vi "AutoAdjustYAlxes.vi"(9 "已选信号数组":refnum<vi>, 10 "YaxleNum":i32, 11 "XYGraph输入":refnum<vi>) -> (1 "显示的Y轴数":i32)   [LabVIEW 2015]
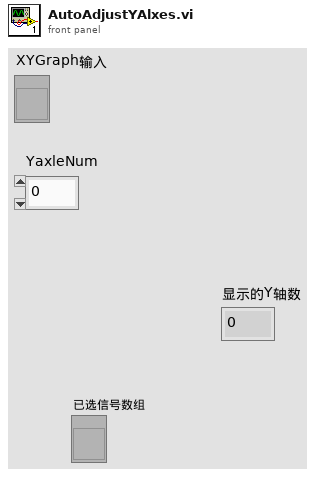
[diagram p1: front panel]
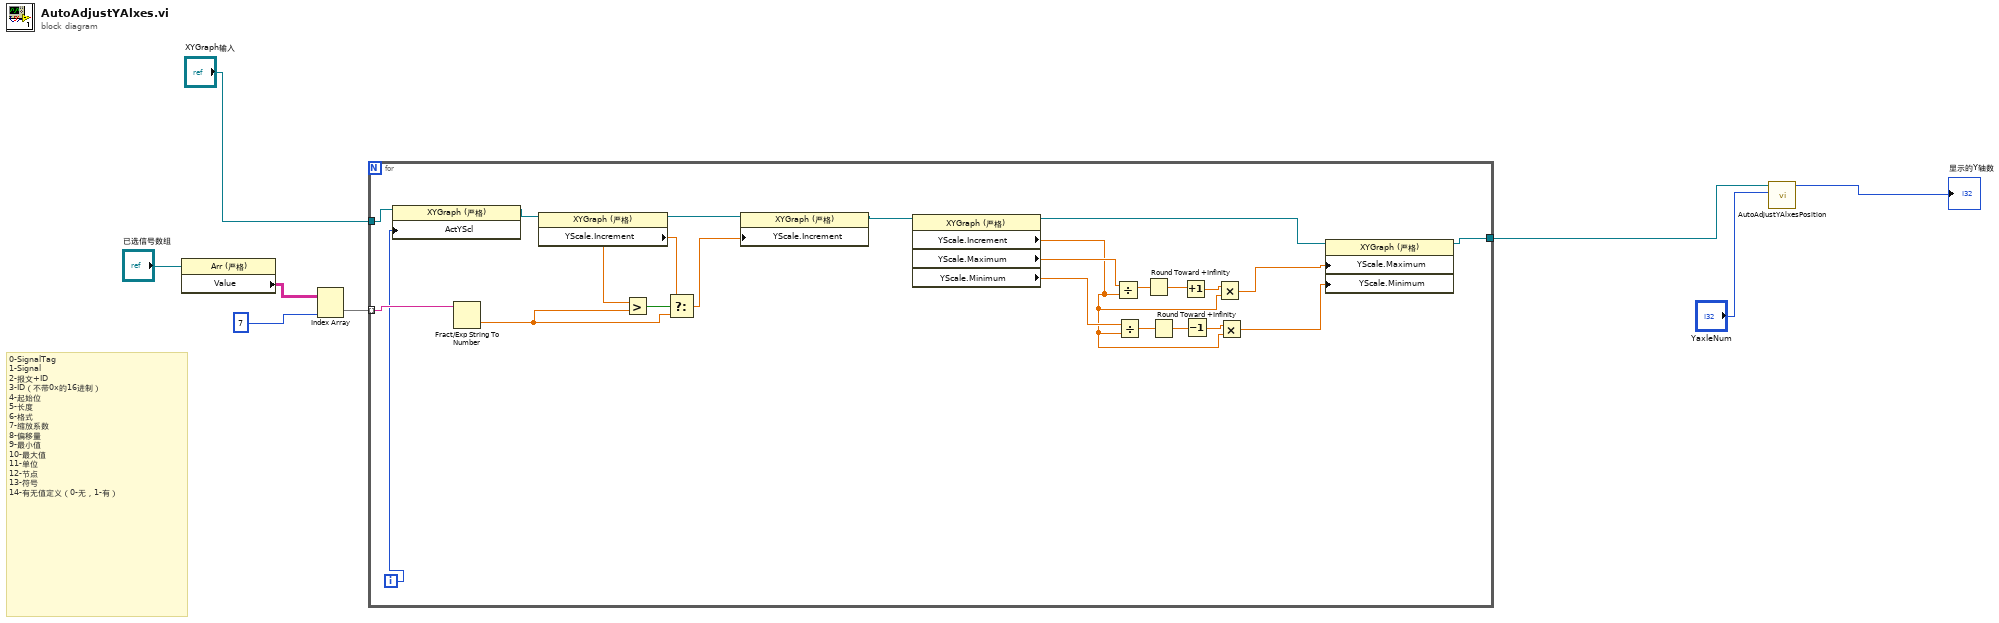
[diagram p0: block diagram]
diagram:
  # "0-SignalTag\n1-Signal\n2-报文+ID\n3-ID（不带0x的16进制）\n4-起始位\n5-长度\n6-格式\n7-缩放系数\n8-偏移量\n9-最小值\n10-最大值\n11-单位\n12-节点\n13-符号\n14-有无值定义（0-无，1-有）"
  n1 = property class="Arr (严格)"(reference="已选信号数组") -> ("Value"=w6:string[][])  [unwired: 1 in, 2 out]
  n2 = Index Array(array=w6, index (col)=7 ("禁用的索引 (列)")) -> (element=w4:string[])  [unwired: 1 in]
  n3 = for {
    tunnel: w4 -> [w31] mode=indexing
    tunnel: "XYGraph输入" -> [w14]
    tunnel: [w16] -> w1
    i -> [w13]
    n4 = property class="XYGraph (严格)"(reference=w14, "ActYScl"=w13) -> (reference out=w15:refnum<vi>)  [unwired: 1 in, 1 out]
    n5 = Fract/Exp String To Number(string=w31) -> (number=w29:dbl)  [unwired: 3 in, 1 out]
    n6 = property class="XYGraph (严格)"(reference=w15) -> (reference out=w11:refnum<vi>, "YScale.Increment"=w26:dbl)  [unwired: 1 in, 1 out]
    n7 = Greater?(x=w26, y=w29) -> (0:w30:bool)
    n8 = Select(t=w26, s=w30, f=w29) -> (s? t:f=w10:dbl)
    n9 = property class="XYGraph (严格)"(reference=w11, "YScale.Increment"=w10) -> (reference out=w12:refnum<vi>)  [unwired: 1 in, 1 out]
    n10 = property class="XYGraph (严格)"(reference=w12) -> (reference out=w17:refnum<vi>, "YScale.Increment"=w9:dbl, "YScale.Maximum"=w22:dbl, "YScale.Minimum"=w25:dbl)  [unwired: 1 in, 1 out]
    n11 = Divide(x=w22, y=w9) -> (x/y=w21:dbl)
    n12 = Divide(x=w25, y=w9) -> (x/y=w27:dbl)
    n13 = Round Toward +Infinity(x=w21) -> (ceil(x): smallest int >= x=w20:dbl)
    n14 = Round Toward +Infinity(x=w27) -> (ceil(x): smallest int >= x=w28:dbl)
    n15 = Increment(x=w20) -> (x+1=w23:dbl)
    n16 = Decrement(x=w28) -> (x-1=w24:dbl)
    n17 = Multiply(x=w23, y=w9) -> (x*y=w19:dbl)
    n18 = Multiply(x=w24, y=w9) -> (x*y=w18:dbl)
    n19 = property class="XYGraph (严格)"(reference=w17, "YScale.Maximum"=w19, "YScale.Minimum"=w18) -> (reference out=w16:refnum<vi>)  [unwired: 1 in, 1 out]
  }
  n20 = call "AutoAdjustYAlxesPosition.vi"("YaxleNum"="YaxleNum", "XYGraph输入"=w1) -> ("显示的Y轴数"=→"显示的Y轴数":i32)  [unwired: 9 in]
